vi "read TBM configuration.vi"(8 "error in":errorcluster, 11 "tag bus configurable plugin editor node in":refnum<class "user tag bus module editor node.lvclass">) -> (0 "error out":errorcluster, 2 "configuration":refnum<class "TBM configuration.lvclass">, 3 "tag bus configurable plugin editor node out":refnum<class "user tag bus module editor node.lvclass">)   [LabVIEW 2013, in "user tag bus module editor node.lvclass"]
uses:
  user tag bus module editor node.lvclass
  <vilib>/NI/Tag Bus Module Framework/root configuration/TBM configuration.lvclass
  user tag bus module editor node.lvclass/user tag bus module editor node.ctl
  module/configuration/user tag bus module configuration.lvclass
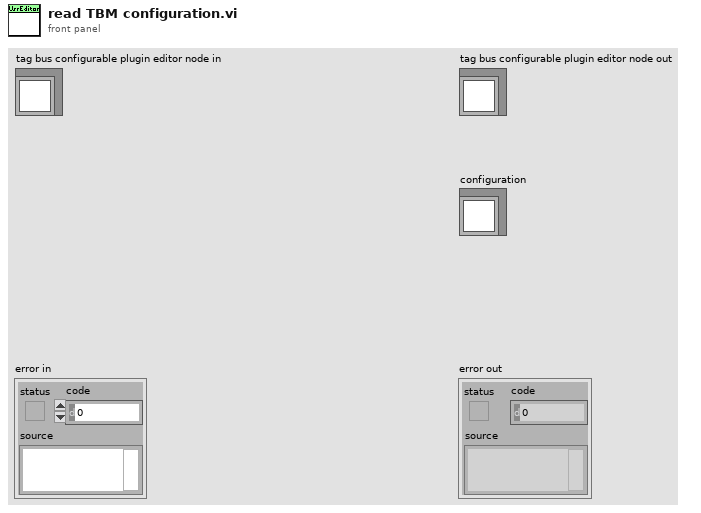
[diagram p1: front panel]
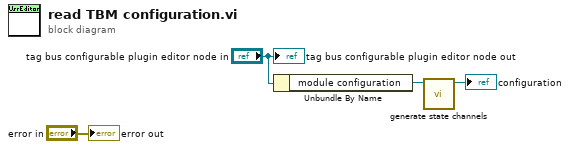
[diagram p0: block diagram]
diagram:
  n1 = Unbundle By Name("tag bus configurable plugin editor node in") -> ("module configuration"=w2:refnum<class "user tag bus module configuration.lvclass">)
  n2 = call "generate state channels.vi"("tag bus configurable plugin module configuration in"=w2) -> ("tag bus configurable plugin module configuration out"=→"configuration":refnum<class "user tag bus module configuration.lvclass">)  [unwired: 9 in, 1 out]
  "error out" <- "error in"
  "tag bus configurable plugin editor node out" <- "tag bus configurable plugin editor node in"
